vi "Parse Decimals.vi"(4 "Format String":string) -> (7 "Decimals":u8)   [LabVIEW 2020, in "VolatusGUIEditorCore.lvlib"]
uses:
  VolatusGUIEditorCore.lvlib
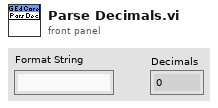
[diagram p1: front panel]
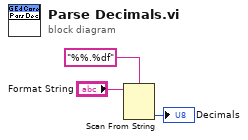
[diagram p0: block diagram]
diagram:
  n1 = Scan From String(format string="%%.%df", input string="Format String") -> (output 1=→"Decimals":u8)  [unwired: 3 in, 3 out]
